vi "Main_14b.vi"() -> ()   [LabVIEW 2020]
uses:
  RB ENUM_Space ID.ctl
  b458f11c-68fc-4924-a47f-25468c26b020.vi
  <vilib>/Comparison/Equal/Equal Functor/Equal Functor.lvclass
panel:
  in  "milliseconds to wait":u32=200
  out "Answer":i32
  out "Sand Path":i32[][](array[numeric])
  in  "Example 2":string="498,4 -> 498,6 -> 496,6\n503,4 -> 502,4 -> 502,9 -> 494,9"
  out "Grid":T1[][](array[typedef])
  in  "Puzzle":string="511,54 -> 511,56 -> 504,56 -> 504,61 -> 520,61 -> 520,56 -> 515,56 -> 515,54\n516,113 -> 521,113\n511,101 -> 511,103 -> 504,103 -> 504,106 -> 517,106 -> 517,103 -> 513,103 -> 513,101\n529,82 -> 533,82\n541,157 -> 545,157\n489,20 -> 489,24 -> 483,24 -> 483,32 -> 495,32 -> 495,24 -> 492,24 -> 492,20\n512,111 -> 517,111\n538,154 -> 542,154\n521,170 -> 521,163 -> 521,170 -> 523,170 -> 523,160 -> 523,170 -> 525,170 -> 525,165 -> 525,170 -> 527,170 -> 527,168 -> 527,170 -> 529,170 -> 529,169 -> 529,170 -> 531,170 -> 531,169 -> 531,170 -> 533,170 -> 533,160 -> 533,170\n521,170 -> 521,163 -> 521,170 -> 523,170 -> 523,160 -> 523,170 -> 525,170 -> 525,165 -> 525,170 -> 527,170 -> 527,168 -> 527,170 -> 529,170 -> 529,169 -> 529,170 -> 531,170 -> 531,169 -> 531,170 -> 533,170 -> 533,160 -> 533,170\n523,76 -> 527,76\n511,101 -> 511,103 -> 504,103 -> 504,106 -> 517,106 -> 517,103 -> 513,103 -> 513,101\n511,82 -> 515,82\n514,79 -> 518,79\n501,98 -> 501,93 -> 501,98 -> 503,98 -> 503,97 -> 503,98 -> 505,98 -> 505,90 -> 505,98 -> 507,98 -> 507,92 -> 507,98 -> 509,98 -> 509,94 -> 509,98 -> 511,98 -> 511,93 -> 511,98\n489,20 -> 489,24 -> 483,24 -> 483,32 -> 495,32 -> 495,24 -> 492,24 -> 492,20\n489,45 -> 489,38 -> 489,45 -> 491,45 -> 491,38 -> 491,45 -> 493,45 -> 493,40 -> 493,45 -> 495,45 -> 495,39 -> 495,45 -> 497,45 -> 497,43 -> 497,45 -> 499,45 -> 499,43 -> 499,45 -> 501,45 -> 501,36 -> 501,45\n501,98 -> 501,93 -> 501,98 -> 503,98 -> 503,97 -> 503,98 -> 505,98 -> 505,90 -> 505,98 -> 507,98 -> 507,92 -> 507,98 -> 509,98 -> 509,94 -> 509,98 -> 511,98 -> 511,93 -> 511,98\n521,170 -> 521,163 -> 521,170 -> 523,170 -> 523,160 -> 523,170 -> 525,170 -> 525,165 -> 525,170 -> 527,170 -> 527,168 -> 527,170 -> 529,170 -> 529,169 -> 529,170 -> 531,170 -> 531,169 -> 531,170 -> 533,170 -> 533,160 -> 533,170\n501,98 -> 501,93 -> 501,98 -> 503,98 -> 503,97 -> 503,98 -> 505,98 -> 505,90 -> 505,98 -> 507,98 -> 507,92 -> 507,98 -> 509,98 -> 509,94 -> 509,98 -> 511,98 -> 511,93 -> 511,98\n514,85 -> 518,85\n528,131 -> 528,121 -> 528,131 -> 530,131 -> 530,127 -> 530,131 -> 532,131 -> 532,124 -> 532,131 -> 534,131 -> 534,126 -> 534,131\n489,45 -> 489,38 -> 489,45 -> 491,45 -> 491,38 -> 491,45 -> 493,45 -> 493,40 -> 493,45 -> 495,45 -> 495,39 -> 495,45 -> 497,45 -> 497,43 -> 497,45 -> 499,45 -> 499,43 -> 499,45 -> 501,45 -> 501,36 -> 501,45\n521,170 -> 521,163 -> 521,170 -> 523,170 -> 523,160 -> 523,170 -> 525,170 -> 525,165 -> 525,170 -> 527,170 -> 527,168 -> 527,170 -> 529,170 -> 529,169 -> 529,170 -> 531,170 -> 531,169 -> 531,170 -> 533,170 -> 533,160 -> 533,170\n489,45 -> 489,38 -> 489,45 -> 491,45 -> 491,38 -> 491,45 -> 493,45 -> 493,40 -> 493,45 -> 495,45 -> 495,39 -> 495,45 -> 497,45 -> 497,43 -> 497,45 -> 499,45 -> 499,43 -> 499,45 -> 501,45 -> 501,36 -> 501,45\n501,98 -> 501,93 -> 501,98 -> 503,98 -> 503,97 -> 503,98 -> 505,98 -> 505,90 -> 505,98 -> 507,98 -> 507,92 -> 507,98 -> 509,98 -> 509,94 -> 509,98 -> 511,98 -> 511,93 -> 511,98\n532,134 -> 532,136 -> 530,136 -> 530,142 -> 542,142 -> 542,136 -> 536,136 -> 536,134\n532,85 -> 536,85\n511,101 -> 511,103 -> 504,103 -> 504,106 -> 517,106 -> 517,103 -> 513,103 -> 513,101\n521,170 -> 521,163 -> 521,170 -> 523,170 -> 523,160 -> 523,170 -> 525,170 -> 525,165 -> 525,170 -> 527,170 -> 527,168 -> 527,170 -> 529,170 -> 529,169 -> 529,170 -> 531,170 -> 531,169 -> 531,170 -> 533,170 -> 533,160 -> 533,170\n528,131 -> 528,121 -> 528,131 -> 530,131 -> 530,127 -> 530,131 -> 532,131 -> 532,124 -> 532,131 -> 534,131 -> 534,126 -> 534,131\n521,170 -> 521,163 -> 521,170 -> 523,170 -> 523,160 -> 523,170 -> 525,170 -> 525,165 -> 525,170 -> 527,170 -> 527,168 -> 527,170 -> 529,170 -> 529,169 -> 529,170 -> 531,170 -> 531,169 -> 531,170 -> 533,170 -> 533,160 -> 533,170\n511,101 -> 511,103 -> 504,103 -> 504,106 -> 517,106 -> 517,103 -> 513,103 -> 513,101\n535,151 -> 539,151\n528,131 -> 528,121 -> 528,131 -> 530,131 -> 530,127 -> 530,131 -> 532,131 -> 532,124 -> 532,131 -> 534,131 -> 534,126 -> 534,131\n501,98 -> 501,93 -> 501,98 -> 503,98 -> 503,97 -> 503,98 -> 505,98 -> 505,90 -> 505,98 -> 507,98 -> 507,92 -> 507,98 -> 509,98 -> 509,94 -> 509,98 -> 511,98 -> 511,93 -> 511,98\n521,170 -> 521,163 -> 521,170 -> 523,170 -> 523,160 -> 523,170 -> 525,170 -> 525,165 -> 525,170 -> 527,170 -> 527,168 -> 527,170 -> 529,170 -> 529,169 -> 529,170 -> 531,170 -> 531,169 -> 531,170 -> 533,170 -> 533,160 -> 533,170\n501,98 -> 501,93 -> 501,98 -> 503,98 -> 503,97 -> 503,98 -> 505,98 -> 505,90 -> 505,98 -> 507,98 -> 507,92 -> 507,98 -> 509,98 -> 509,94 -> 509,98 -> 511,98 -> 511,93 -> 511,98\n501,98 -> 501,93 -> 501,98 -> 503,98 -> 503,97 -> 503,98 -> 505,98 -> 505,90 -> 505,98 -> 507,98 -> 507,92 -> 507,98 -> 509,98 -> 509,94 -> 509,98 -> 511,98 -> 511,93 -> 511,98\n526,85 -> 530,85\n497,50 -> 497,51 -> 512,51\n532,134 -> 532,136 -> 530,136 -> 530,142 -> 542,142 -> 542,136 -> 536,136 -> 536,134\n501,98 -> 501,93 -> 501,98 -> 503,98 -> 503,97 -> 503,98 -> 505,98 -> 505,90 -> 505,98 -> 507,98 -> 507,92 -> 507,98 -> 509,98 -> 509,94 -> 509,98 -> 511,98 -> 511,93 -> 511,98\n489,45 -> 489,38 -> 489,45 -> 491,45 -> 491,38 -> 491,45 -> 493,45 -> 493,40 -> 493,45 -> 495,45 -> 495,39 -> 495,45 -> 497,45 -> 497,43 -> 497,45 -> 499,45 -> 499,43 -> 499,45 -> 501,45 -> 501,36 -> 501,45\n509,113 -> 514,113\n489,45 -> 489,38 -> 489,45 -> 491,45 -> 491,38 -> 491,45 -> 493,45 -> 493,40 -> 493,45 -> 495,45 -> 495,39 -> 495,45 -> 497,45 -> 497,43 -> 497,45 -> 499,45 -> 499,43 -> 499,45 -> 501,45 -> 501,36 -> 501,45\n489,45 -> 489,38 -> 489,45 -> 491,45 -> 491,38 -> 491,45 -> 493,45 -> 493,40 -> 493,45 -> 495,45 -> 495,39 -> 495,45 -> 497,45 -> 497,43 -> 497,45 -> 499,45 -> 499,43 -> 499,45 -> 501,45 -> 501,36 -> 501,45\n538,148 -> 542,148\n492,17 -> 496,17\n521,170 -> 521,163 -> 521,170 -> 523,170 -> 523,160 -> 523,170 -> 525,170 -> 525,165 -> 525,170 -> 527,170 -> 527,168 -> 527,170 -> 529,170 -> 529,169 -> 529,170 -> 531,170 -> 531,169 -> 531,170 -> 533,170 -> 533,160 -> 533,170\n528,131 -> 528,121 -> 528,131 -> 530,131 -> 530,127 -> 530,131 -> 532,131 -> 532,124 -> 532,131 -> 534,131 -> 534,126 -> 534,131\n489,45 -> 489,38 -> 489,45 -> 491,45 -> 491,38 -> 491,45 -> 493,45 -> 493,40 -> 493,45 -> 495,45 -> 495,39 -> 495,45 -> 497,45 -> 497,43 -> 497,45 -> 499,45 -> 499,43 -> 499,45 -> 501,45 -> 501,36 -> 501,45\n511,54 -> 511,56 -> 504,56 -> 504,61 -> 520,61 -> 520,56 -> 515,56 -> 515,54\n541,145 -> 545,145\n497,50 -> 497,51 -> 512,51\n501,98 -> 501,93 -> 501,98 -> 503,98 -> 503,97 -> 503,98 -> 505,98 -> 505,90 -> 505,98 -> 507,98 -> 507,92 -> 507,98 -> 509,98 -> 509,94 -> 509,98 -> 511,98 -> 511,93 -> 511,98\n550,154 -> 554,154\n521,170 -> 521,163 -> 521,170 -> 523,170 -> 523,160 -> 523,170 -> 525,170 -> 525,165 -> 525,170 -> 527,170 -> 527,168 -> 527,170 -> 529,170 -> 529,169 -> 529,170 -> 531,170 -> 531,169 -> 531,170 -> 533,170 -> 533,160 -> 533,170\n520,79 -> 524,79\n489,45 -> 489,38 -> 489,45 -> 491,45 -> 491,38 -> 491,45 -> 493,45 -> 493,40 -> 493,45 -> 495,45 -> 495,39 -> 495,45 -> 497,45 -> 497,43 -> 497,45 -> 499,45 -> 499,43 -> 499,45 -> 501,45 -> 501,36 -> 501,45\n517,63 -> 517,64 -> 524,64 -> 524,63\n489,20 -> 489,24 -> 483,24 -> 483,32 -> 495,32 -> 495,24 -> 492,24 -> 492,20\n532,154 -> 536,154\n489,20 -> 489,24 -> 483,24 -> 483,32 -> 495,32 -> 495,24 -> 492,24 -> 492,20\n489,45 -> 489,38 -> 489,45 -> 491,45 -> 491,38 -> 491,45 -> 493,45 -> 493,40 -> 493,45 -> 495,45 -> 495,39 -> 495,45 -> 497,45 -> 497,43 -> 497,45 -> 499,45 -> 499,43 -> 499,45 -> 501,45 -> 501,36 -> 501,45\n501,98 -> 501,93 -> 501,98 -> 503,98 -> 503,97 -> 503,98 -> 505,98 -> 505,90 -> 505,98 -> 507,98 -> 507,92 -> 507,98 -> 509,98 -> 509,94 -> 509,98 -> 511,98 -> 511,93 -> 511,98\n521,117 -> 521,118 -> 531,118 -> 531,117\n528,131 -> 528,121 -> 528,131 -> 530,131 -> 530,127 -> 530,131 -> 532,131 -> 532,124 -> 532,131 -> 534,131 -> 534,126 -> 534,131\n532,134 -> 532,136 -> 530,136 -> 530,142 -> 542,142 -> 542,136 -> 536,136 -> 536,134\n501,98 -> 501,93 -> 501,98 -> 503,98 -> 503,97 -> 503,98 -> 505,98 -> 505,90 -> 505,98 -> 507,98 -> 507,92 -> 507,98 -> 509,98 -> 509,94 -> 509,98 -> 511,98 -> 511,93 -> 511,98\n547,157 -> 551,157\n532,134 -> 532,136 -> 530,136 -> 530,142 -> 542,142 -> 542,136 -> 536,136 -> 536,134\n521,117 -> 521,118 -> 531,118 -> 531,117\n517,63 -> 517,64 -> 524,64 -> 524,63\n501,98 -> 501,93 -> 501,98 -> 503,98 -> 503,97 -> 503,98 -> 505,98 -> 505,90 -> 505,98 -> 507,98 -> 507,92 -> 507,98 -> 509,98 -> 509,94 -> 509,98 -> 511,98 -> 511,93 -> 511,98\n521,170 -> 521,163 -> 521,170 -> 523,170 -> 523,160 -> 523,170 -> 525,170 -> 525,165 -> 525,170 -> 527,170 -> 527,168 -> 527,170 -> 529,170 -> 529,169 -> 529,170 -> 531,170 -> 531,169 -> 531,170 -> 533,170 -> 533,160 -> 533,170\n523,82 -> 527,82\n489,45 -> 489,38 -> 489,45 -> 491,45 -> 491,38 -> 491,45 -> 493,45 -> 493,40 -> 493,45 -> 495,45 -> 495,39 -> 495,45 -> 497,45 -> 497,43 -> 497,45 -> 499,45 -> 499,43 -> 499,45 -> 501,45 -> 501,36 -> 501,45\n495,15 -> 499,15\n553,157 -> 557,157\n511,101 -> 511,103 -> 504,103 -> 504,106 -> 517,106 -> 517,103 -> 513,103 -> 513,101\n498,17 -> 502,17\n528,131 -> 528,121 -> 528,131 -> 530,131 -> 530,127 -> 530,131 -> 532,131 -> 532,124 -> 532,131 -> 534,131 -> 534,126 -> 534,131\n532,134 -> 532,136 -> 530,136 -> 530,142 -> 542,142 -> 542,136 -> 536,136 -> 536,134\n521,170 -> 521,163 -> 521,170 -> 523,170 -> 523,160 -> 523,170 -> 525,170 -> 525,165 -> 525,170 -> 527,170 -> 527,168 -> 527,170 -> 529,170 -> 529,169 -> 529,170 -> 531,170 -> 531,169 -> 531,170 -> 533,170 -> 533,160 -> 533,170\n547,151 -> 551,151\n521,170 -> 521,163 -> 521,170 -> 523,170 -> 523,160 -> 523,170 -> 525,170 -> 525,165 -> 525,170 -> 527,170 -> 527,168 -> 527,170 -> 529,170 -> 529,169 -> 529,170 -> 531,170 -> 531,169 -> 531,170 -> 533,170 -> 533,160 -> 533,170\n511,101 -> 511,103 -> 504,103 -> 504,106 -> 517,106 -> 517,103 -> 513,103 -> 513,101\n504,17 -> 508,17\n544,148 -> 548,148\n521,170 -> 521,163 -> 521,170 -> 523,170 -> 523,160 -> 523,170 -> 525,170 -> 525,165 -> 525,170 -> 527,170 -> 527,168 -> 527,170 -> 529,170 -> 529,169 -> 529,170 -> 531,170 -> 531,169 -> 531,170 -> 533,170 -> 533,160 -> 533,170\n511,54 -> 511,56 -> 504,56 -> 504,61 -> 520,61 -> 520,56 -> 515,56 -> 515,54\n489,45 -> 489,38 -> 489,45 -> 491,45 -> 491,38 -> 491,45 -> 493,45 -> 493,40 -> 493,45 -> 495,45 -> 495,39 -> 495,45 -> 497,45 -> 497,43 -> 497,45 -> 499,45 -> 499,43 -> 499,45 -> 501,45 -> 501,36 -> 501,45\n489,45 -> 489,38 -> 489,45 -> 491,45 -> 491,38 -> 491,45 -> 493,45 -> 493,40 -> 493,45 -> 495,45 -> 495,39 -> 495,45 -> 497,45 -> 497,43 -> 497,45 -> 499,45 -> 499,43 -> 499,45 -> 501,45 -> 501,36 -> 501,45\n489,45 -> 489,38 -> 489,45 -> 491,45 -> 491,38 -> 491,45 -> 493,45 -> 493,40 -> 493,45 -> 495,45 -> 495,39 -> 495,45 -> 497,45 -> 497,43 -> 497,45 -> 499,45 -> 499,43 -> 499,45 -> 501,45 -> 501,36 -> 501,45\n523,113 -> 528,113\n521,170 -> 521,163 -> 521,170 -> 523,170 -> 523,160 -> 523,170 -> 525,170 -> 525,165 -> 525,170 -> 527,170 -> 527,168 -> 527,170 -> 529,170 -> 529,169 -> 529,170 -> 531,170 -> 531,169 -> 531,170 -> 533,170 -> 533,160 -> 533,170\n535,157 -> 539,157\n521,170 -> 521,163 -> 521,170 -> 523,170 -> 523,160 -> 523,170 -> 525,170 -> 525,165 -> 525,170 -> 527,170 -> 527,168 -> 527,170 -> 529,170 -> 529,169 -> 529,170 -> 531,170 -> 531,169 -> 531,170 -> 533,170 -> 533,160 -> 533,170\n528,131 -> 528,121 -> 528,131 -> 530,131 -> 530,127 -> 530,131 -> 532,131 -> 532,124 -> 532,131 -> 534,131 -> 534,126 -> 534,131\n489,45 -> 489,38 -> 489,45 -> 491,45 -> 491,38 -> 491,45 -> 493,45 -> 493,40 -> 493,45 -> 495,45 -> 495,39 -> 495,45 -> 497,45 -> 497,43 -> 497,45 -> 499,45 -> 499,43 -> 499,45 -> 501,45 -> 501,36 -> 501,45\n521,170 -> 521,163 -> 521,170 -> 523,170 -> 523,160 -> 523,170 -> 525,170 -> 525,165 -> 525,170 -> 527,170 -> 527,168 -> 527,170 -> 529,170 -> 529,169 -> 529,170 -> 531,170 -> 531,169 -> 531,170 -> 533,170 -> 533,160 -> 533,170\n521,170 -> 521,163 -> 521,170 -> 523,170 -> 523,160 -> 523,170 -> 525,170 -> 525,165 -> 525,170 -> 527,170 -> 527,168 -> 527,170 -> 529,170 -> 529,169 -> 529,170 -> 531,170 -> 531,169 -> 531,170 -> 533,170 -> 533,160 -> 533,170\n498,13 -> 502,13\n532,134 -> 532,136 -> 530,136 -> 530,142 -> 542,142 -> 542,136 -> 536,136 -> 536,134\n526,79 -> 530,79\n511,54 -> 511,56 -> 504,56 -> 504,61 -> 520,61 -> 520,56 -> 515,56 -> 515,54\n511,54 -> 511,56 -> 504,56 -> 504,61 -> 520,61 -> 520,56 -> 515,56 -> 515,54\n521,117 -> 521,118 -> 531,118 -> 531,117\n541,151 -> 545,151\n501,98 -> 501,93 -> 501,98 -> 503,98 -> 503,97 -> 503,98 -> 505,98 -> 505,90 -> 505,98 -> 507,98 -> 507,92 -> 507,98 -> 509,98 -> 509,94 -> 509,98 -> 511,98 -> 511,93 -> 511,98\n489,45 -> 489,38 -> 489,45 -> 491,45 -> 491,38 -> 491,45 -> 493,45 -> 493,40 -> 493,45 -> 495,45 -> 495,39 -> 495,45 -> 497,45 -> 497,43 -> 497,45 -> 499,45 -> 499,43 -> 499,45 -> 501,45 -> 501,36 -> 501,45\n532,134 -> 532,136 -> 530,136 -> 530,142 -> 542,142 -> 542,136 -> 536,136 -> 536,134\n501,98 -> 501,93 -> 501,98 -> 503,98 -> 503,97 -> 503,98 -> 505,98 -> 505,90 -> 505,98 -> 507,98 -> 507,92 -> 507,98 -> 509,98 -> 509,94 -> 509,98 -> 511,98 -> 511,93 -> 511,98\n489,20 -> 489,24 -> 483,24 -> 483,32 -> 495,32 -> 495,24 -> 492,24 -> 492,20\n519,111 -> 524,111\n489,45 -> 489,38 -> 489,45 -> 491,45 -> 491,38 -> 491,45 -> 493,45 -> 493,40 -> 493,45 -> 495,45 -> 495,39 -> 495,45 -> 497,45 -> 497,43 -> 497,45 -> 499,45 -> 499,43 -> 499,45 -> 501,45 -> 501,36 -> 501,45\n529,157 -> 533,157\n511,101 -> 511,103 -> 504,103 -> 504,106 -> 517,106 -> 517,103 -> 513,103 -> 513,101\n501,15 -> 505,15\n528,131 -> 528,121 -> 528,131 -> 530,131 -> 530,127 -> 530,131 -> 532,131 -> 532,124 -> 532,131 -> 534,131 -> 534,126 -> 534,131\n489,20 -> 489,24 -> 483,24 -> 483,32 -> 495,32 -> 495,24 -> 492,24 -> 492,20\n508,85 -> 512,85\n520,85 -> 524,85\n489,45 -> 489,38 -> 489,45 -> 491,45 -> 491,38 -> 491,45 -> 493,45 -> 493,40 -> 493,45 -> 495,45 -> 495,39 -> 495,45 -> 497,45 -> 497,43 -> 497,45 -> 499,45 -> 499,43 -> 499,45 -> 501,45 -> 501,36 -> 501,45\n517,76 -> 521,76\n517,82 -> 521,82\n489,45 -> 489,38 -> 489,45 -> 491,45 -> 491,38 -> 491,45 -> 493,45 -> 493,40 -> 493,45 -> 495,45 -> 495,39 -> 495,45 -> 497,45 -> 497,43 -> 497,45 -> 499,45 -> 499,43 -> 499,45 -> 501,45 -> 501,36 -> 501,45\n523,69 -> 523,70 -> 530,70\n520,73 -> 524,73\n528,131 -> 528,121 -> 528,131 -> 530,131 -> 530,127 -> 530,131 -> 532,131 -> 532,124 -> 532,131 -> 534,131 -> 534,126 -> 534,131\n544,154 -> 548,154\n511,54 -> 511,56 -> 504,56 -> 504,61 -> 520,61 -> 520,56 -> 515,56 -> 515,54\n511,54 -> 511,56 -> 504,56 -> 504,61 -> 520,61 -> 520,56 -> 515,56 -> 515,54\n489,45 -> 489,38 -> 489,45 -> 491,45 -> 491,38 -> 491,45 -> 493,45 -> 493,40 -> 493,45 -> 495,45 -> 495,39 -> 495,45 -> 497,45 -> 497,43 -> 497,45 -> 499,45 -> 499,43 -> 499,45 -> 501,45 -> 501,36 -> 501,45\n501,98 -> 501,93 -> 501,98 -> 503,98 -> 503,97 -> 503,98 -> 505,98 -> 505,90 -> 505,98 -> 507,98 -> 507,92 -> 507,98 -> 509,98 -> 509,94 -> 509,98 -> 511,98 -> 511,93 -> 511,98\n515,109 -> 520,109\n521,170 -> 521,163 -> 521,170 -> 523,170 -> 523,160 -> 523,170 -> 525,170 -> 525,165 -> 525,170 -> 527,170 -> 527,168 -> 527,170 -> 529,170 -> 529,169 -> 529,170 -> 531,170 -> 531,169 -> 531,170 -> 533,170 -> 533,160 -> 533,170\n517,63 -> 517,64 -> 524,64 -> 524,63\n528,131 -> 528,121 -> 528,131 -> 530,131 -> 530,127 -> 530,131 -> 532,131 -> 532,124 -> 532,131 -> 534,131 -> 534,126 -> 534,131\n501,98 -> 501,93 -> 501,98 -> 503,98 -> 503,97 -> 503,98 -> 505,98 -> 505,90 -> 505,98 -> 507,98 -> 507,92 -> 507,98 -> 509,98 -> 509,94 -> 509,98 -> 511,98 -> 511,93 -> 511,98\n521,170 -> 521,163 -> 521,170 -> 523,170 -> 523,160 -> 523,170 -> 525,170 -> 525,165 -> 525,170 -> 527,170 -> 527,168 -> 527,170 -> 529,170 -> 529,169 -> 529,170 -> 531,170 -> 531,169 -> 531,170 -> 533,170 -> 533,160 -> 533,170\n523,69 -> 523,70 -> 530,70\n528,131 -> 528,121 -> 528,131 -> 530,131 -> 530,127 -> 530,131 -> 532,131 -> 532,124 -> 532,131 -> 534,131 -> 534,126 -> 534,131\n501,98 -> 501,93 -> 501,98 -> 503,98 -> 503,97 -> 503,98 -> 505,98 -> 505,90 -> 505,98 -> 507,98 -> 507,92 -> 507,98 -> 509,98 -> 509,94 -> 509,98 -> 511,98 -> 511,93 -> 511,98\n489,45 -> 489,38 -> 489,45 -> 491,45 -> 491,38 -> 491,45 -> 493,45 -> 493,40 -> 493,45 -> 495,45 -> 495,39 -> 495,45 -> 497,45 -> 497,43 -> 497,45 -> 499,45 -> 499,43 -> 499,45 -> 501,45 -> 501,36 -> 501,45\n489,20 -> 489,24 -> 483,24 -> 483,32 -> 495,32 -> 495,24 -> 492,24 -> 492,20\n521,170 -> 521,163 -> 521,170 -> 523,170 -> 523,160 -> 523,170 -> 525,170 -> 525,165 -> 525,170 -> 527,170 -> 527,168 -> 527,170 -> 529,170 -> 529,169 -> 529,170 -> 531,170 -> 531,169 -> 531,170 -> 533,170 -> 533,160 -> 533,170"
  in  "Example":string="498,4 -> 498,6 -> 496,6\n503,4 -> 502,4 -> 502,9 -> 494,9"
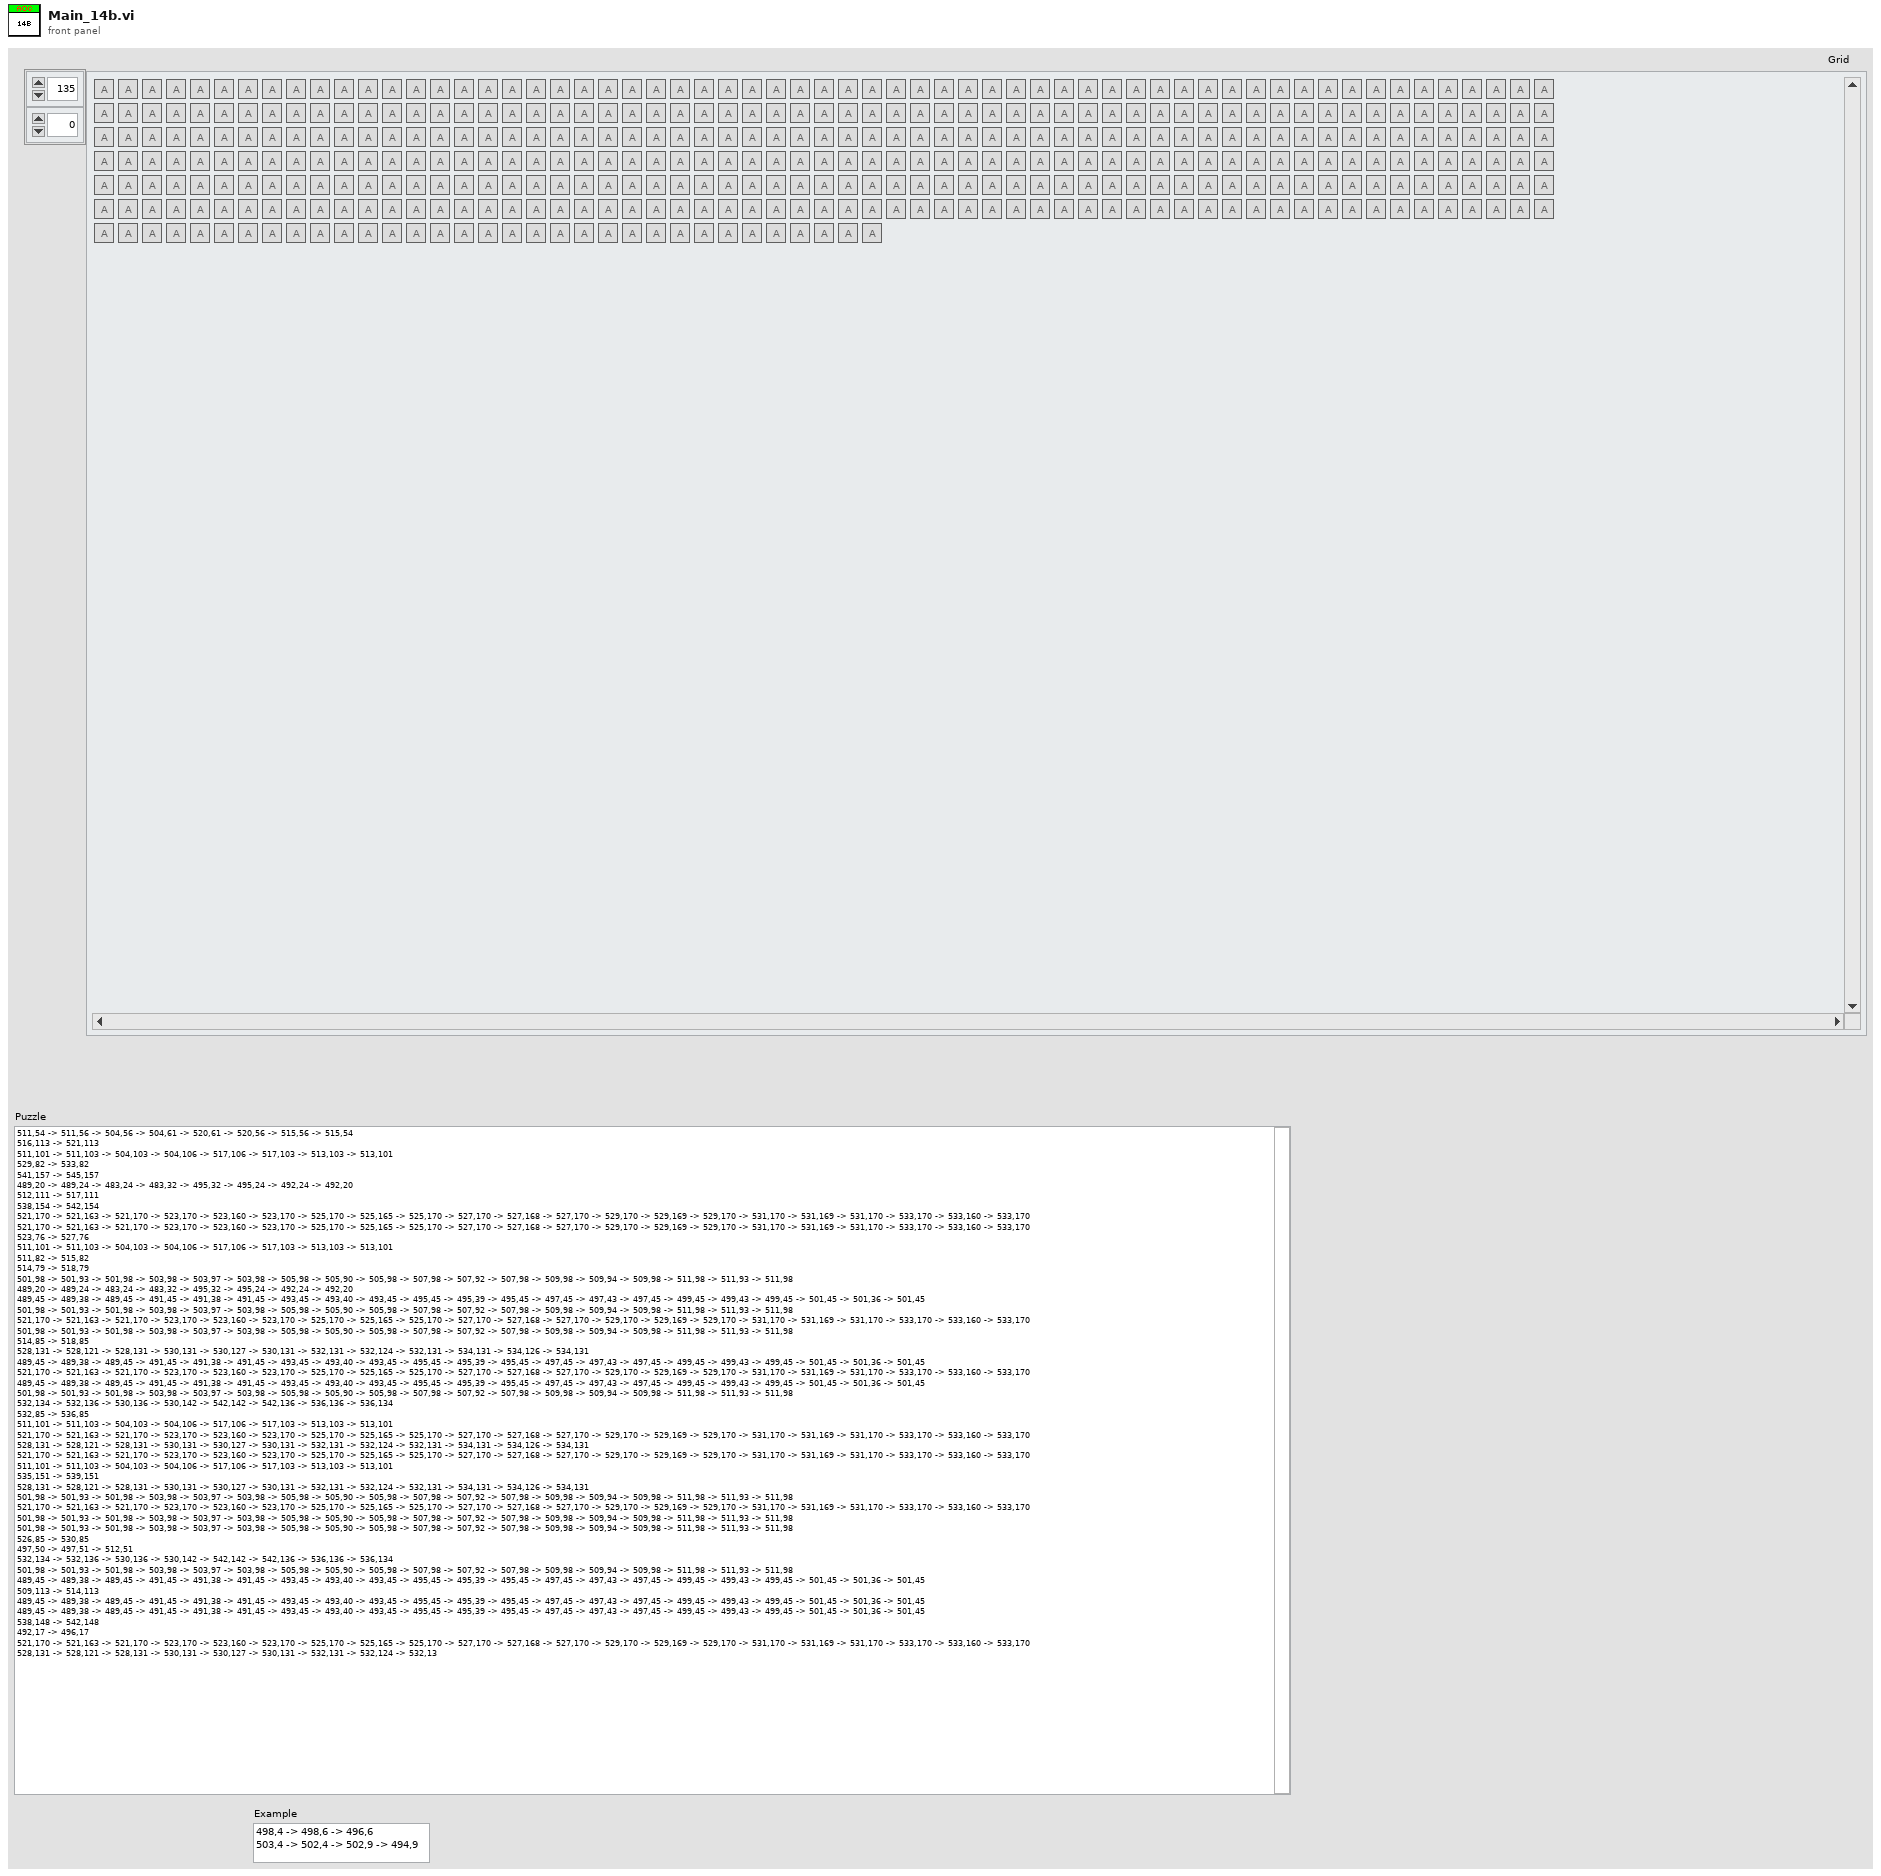
[diagram p1: front panel]
types:
  T1 = typedef "RB ENUM_Space ID.ctl" = enum32{"Air", "Sand", "Rock", "Start", "Abyss"}
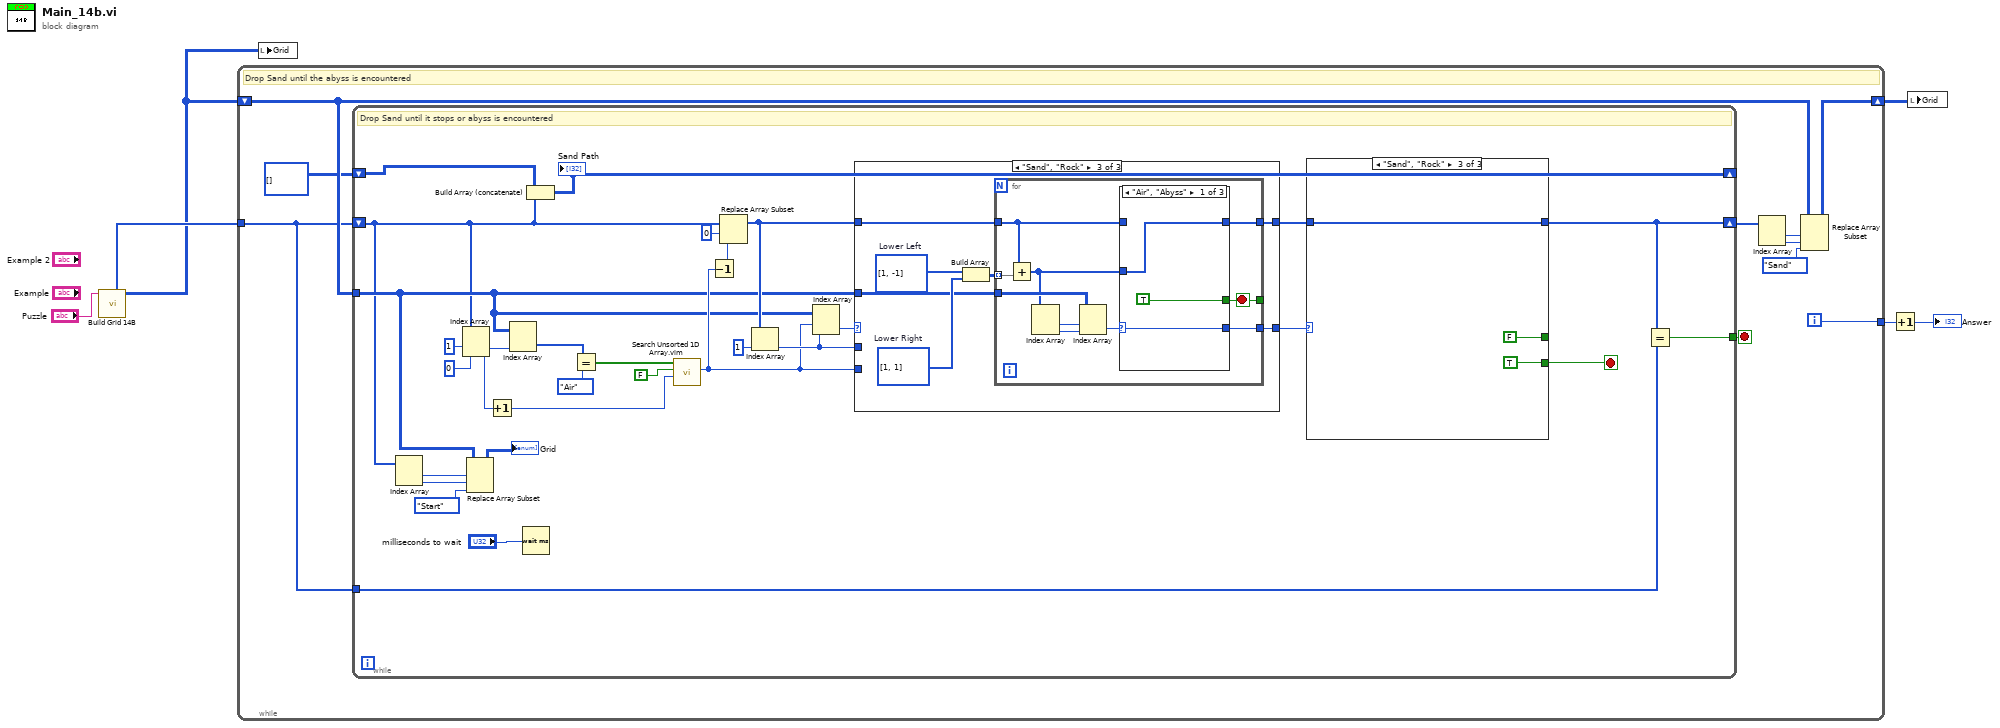
[diagram p0: block diagram]
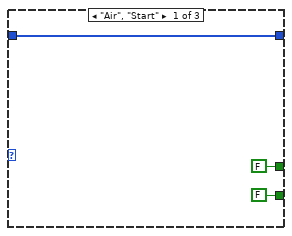
[diagram p2: hidden frame]
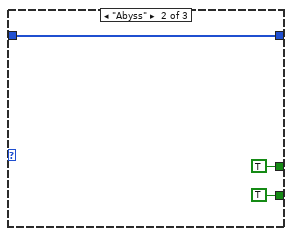
[diagram p3: hidden frame]
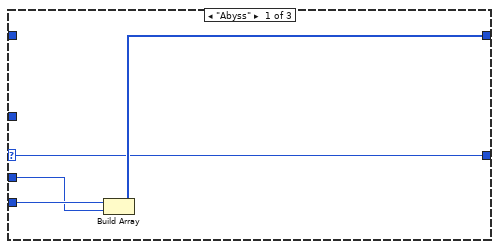
[diagram p4: hidden frame]
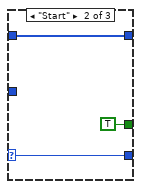
[diagram p6: hidden frame]
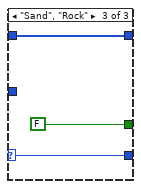
[diagram p7: hidden frame]
diagram:
  n1 = call "Build Grid 14B.vi"("Text"="Puzzle") -> ("Array"=w5:T1[][], "Start"=w6:i32[])  [unwired: 8 in, 1 out]
  n2 = while {
    shift-right: [w11] -> w3
    shift-left: w5 -> [w10]
    tunnel: w6 -> [w7]
    tunnel: [w8] -> w4
    i -> [w8]
    stop <- w12 stop-if-true
    # "Drop Sand until the abyss is encountered"
    n3 = while {
      shift-right: [w20] -> w16
      shift-left: w7 -> [w19]
      tunnel: w10 -> [w26]
      tunnel: [w18] -> w12
      shift-right: [w29] -> _
      shift-left: i32[][] [] -> [w30]
      tunnel: w7 -> [w17]
      stop <- w32 stop-if-true
      # "Drop Sand until it stops or abyss is encountered"
      n4 = Index Array(array=w19) -> (element #1=w24:i32, element #2=w23:i32)  [unwired: 2 in]
      n5 = Index Array(array=w19, index #1=1 ("index"), index #2=0 ("index")) -> (element #1=w46:i32, element #2=w27:i32)
      n6 = Replace Array Subset(array=w26, new element=RB_ENUM_Space_ID."Start" ("new element/subarray"), index (row)=w24, index (col)=w23) -> (→"Grid":T1[][])
      n7 = Increment(x=w27) -> (x+1=w44:i32)
      n8 = Index Array(array=w26, index (col)=w46) -> (element=w45:T1[])  [unwired: 1 in]
      n9 = Wait (ms)(milliseconds to wait="milliseconds to wait") -> ()  [unwired: 1 out]
      n10 = Build Array (concatenate)(w30, w19) -> (w29:i32[][])
      "Sand Path" <- w29
      n11 = Equal?(x=w45, y=RB_ENUM_Space_ID."Air" ("new element/subarray")) -> (x = y?=w42:bool[])
      n12 = call "Search Unsorted 1D Array.vim"("start index (0)"=w44, "element"=FALSE, "unsorted 1D array"=w42) -> ("index of element"=w34:i32)  [unwired: 8 in]
      n13 = Decrement(x=w34) -> (x-1=w39:i32)
      n14 = Replace Array Subset(array=w19, new element=w39, index=0) -> (w36:i32[])
      n15 = Index Array(array=w36, index=1) -> (element=w35:i32)
      n16 = Index Array(array=w26, index (row)=w34, index (col)=w35) -> (element=w37:T1)
      n17 = case shown="\"Sand\", \"Rock\"" w37 {
        selector: w37 -> [w57 w62 _]
        tunnel: w36 -> [_ w61 w66]
        tunnel: w26 -> [_ _ w65]
        tunnel: [w57 w62 w64] -> w33
        tunnel: [w58 w61 w63] -> w31
        tunnel: w35 -> [w59 _ _]
        tunnel: w34 -> [w60 _ _]
        frame "Abyss" {
          n18 = Build Array(w60, w59) -> (w58:i32[])
        }
        frame "Air", "Start" {
          # "Problem if you get here"
        }
        frame "Sand", "Rock" {
          w68 = i32[] [1, 1]  # Lower Right
          w69 = i32[] [1, -1]  # Lower Left
          n19 = Build Array(w69, w68) -> (w67:i32[][])
          n20 = for {
            tunnel: w67 -> [w79] mode=indexing
            tunnel: w66 -> [w70]
            tunnel: w65 -> [w77]
            tunnel: [w73] -> w63
            tunnel: [w72] -> _
            tunnel: [w71] -> w64
            stop <- w72 stop-if-true
            n21 = Add(x=w70, y=w79) -> (x+y=w74:i32[])
            n22 = Index Array(array=w74) -> (element #1=w78:i32, element #2=w76:i32)  [unwired: 2 in]
            n23 = Index Array(array=w77, index (row)=w78, index (col)=w76) -> (element=w75:T1)
            n24 = case shown="\"Air\", \"Abyss\"" w75 {
              selector: w75 -> [w80 w83 w87]
              tunnel: w74 -> [w82 _ _]
              tunnel: [w82 w85 w88] -> w73
              tunnel: [TRUE TRUE FALSE] -> w72
              tunnel: [w80 w83 w87] -> w71
              tunnel: w70 -> [_ w85 w88]
              frame "Air", "Abyss" {
              }
              frame "Start" {
              }
              frame "Sand", "Rock" {
              }
            }
          }
        }
      }
      n25 = case shown="\"Sand\", \"Rock\"" w33 {
        tunnel: [FALSE TRUE TRUE] -> w32
        tunnel: w31 -> [w50 w53 w55]
        tunnel: [w50 w53 w55] -> w20
        tunnel: [FALSE TRUE FALSE] -> _
        frame "Air", "Start" {
        }
        frame "Abyss" {
        }
        frame "Sand", "Rock" {
        }
      }
      n26 = Equal?(x=w20, y=w17) -> (x = y?=w18:bool)
    }
    n27 = Index Array(array=w16) -> (element #1=w14:i32, element #2=w15:i32)  [unwired: 2 in]
    n28 = Replace Array Subset(array=w10, new element=RB_ENUM_Space_ID."Sand" ("new element/subarray"), index (row)=w14, index (col)=w15) -> (w11:T1[][])
  }
  n29 = local write "Grid"(w5) -> ()
  n30 = Increment(x=w4) -> (x+1=→"Answer":i32)
  n31 = local write "Grid"(w3) -> ()
